vi "Trawnik_zmienne.vi"() -> ()   [LabVIEW 2023]
panel:
  in  "Czas podlewania":dbl
  in  "Liczba zraszaczy":dbl
  in  "Powierzchnia":dbl
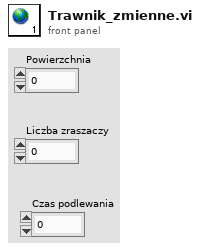
[diagram p1: front panel]
diagram:
